vi "Set Cell Alignment.vi"(1 "Vertical alignment":T1, 4 "Horizontal alignment":T2, 5 "Text Rotation":i32 min=0 max=180 step=1, 6 "error in (no error)":errorcluster, 7 "End Cell Address":string, 8 "Wrap Text":bool, 9 "Start Cell Address":string, 10 "Report Ref In":T3) -> (0 "error out":errorcluster, 3 "Report Ref Out":T3)   [LabVIEW 2013, in "XCel Report Engine.lvlib"]
doc: "Applies text alignment settings to a cell or rectangular cell range in the active worksheet.\n\nStart Cell Address and End Cell Address use Excel A1 notation. If End Cell Address is empty, formatting is applied only to Start Cell Address.\n\nHorizontal Alignment and Vertical Alignment control the position of the cell contents. Wrap Text enables text wrapping within the cell, and Text Rotation specifies the text orientation using a value from 0 to 180.\n\nThe operation preserves cell values, formulas, and unrelated formatting properties.\n\nAn error is returned if either cell address is invalid, the end cell precedes the start cell, or Text Rotation is outside the supported range."
uses:
  XCel Report Engine.lvlib
  C:/Users/m.santucci/Documents/ChatGPT/LV_REPORT_ENGINE/LV/DotNet/XCelReportEngine.dll
  LV/DotNet/XCelReportEngine.dll
  Controls/Report Ref.ctl
  Controls/Horizontal alignment.ctl
  Controls/Vertical alignment.ctl
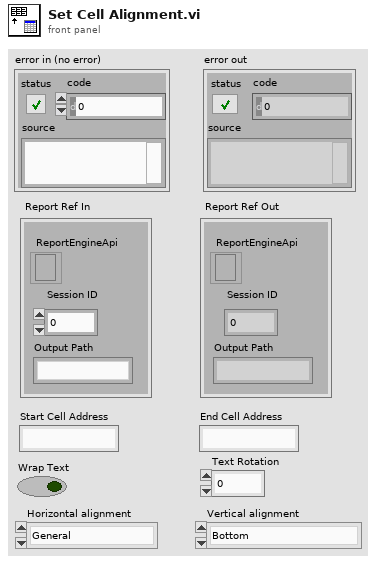
[diagram p1: front panel]
types:
  T1 = typedef "XCel Report Engine.lvlib/Vertical alignment.ctl" = enum16{"Bottom", "Center", "Top", "Justify", "Distributed"}
  T2 = typedef "XCel Report Engine.lvlib/Horizontal alignment.ctl" = enum16{"General", "Left", "Center", "Right", "Fill", "Justify", "CenterContinuous", "Distributed"}
  T3 = typedef "XCel Report Engine.lvlib/Report Ref.ctl" = cluster{"Session ID":i32, "Output Path":string, "ReportEngineApi":refnum<k24>}
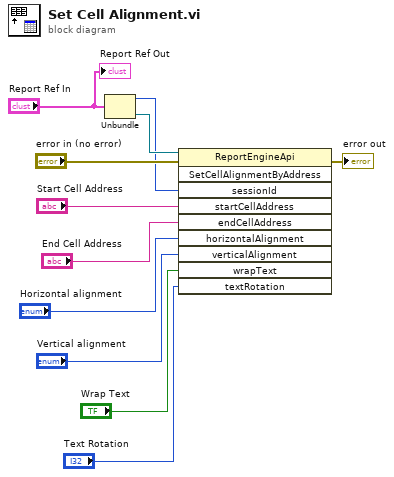
[diagram p0: block diagram]
diagram:
  n1 = Unbundle("Report Ref In") -> ("Session ID"=w7:i32, "ReportEngineApi"=w10:refnum<k24>)  [unwired: 1 out]
  n2 = invoke class="ReportEngineApi" method="SetCellAlignmentByAddress"(reference=w10, error in="error in (no error)", "sessionId"=w7, "startCellAddress"="Start Cell Address", "endCellAddress"="End Cell Address", "horizontalAlignment"="Horizontal alignment", "verticalAlignment"="Vertical alignment", "wrapText"="Wrap Text", "textRotation"="Text Rotation") -> (error out=→"error out":errorcluster)  [unwired: 1 in, 9 out]
  "Report Ref Out" <- "Report Ref In"
